vi "random_bit_sequence.vi"(11 "Length":i32) -> (3 "Bit Sequence":i8[](array[numeric]))   [LabVIEW 2012]
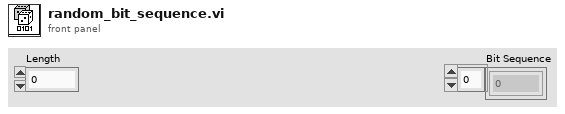
[diagram p1: front panel]
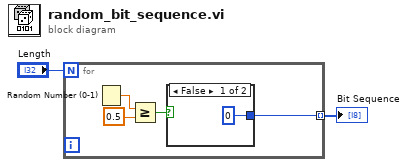
[diagram p0: block diagram]
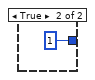
[diagram p2: hidden frame]
diagram:
  n1 = for {
    N: "Length" -> [_]
    tunnel: [w3] -> w1 mode=indexing
    n2 = Random Number (0-1)() -> (number: 0 to 1=w5:dbl)
    n3 = Greater Or Equal?(x=w5, y=0.5) -> (x >= y?=w4:bool)
    n4 = case shown="False" w4 {
      tunnel: [i8 0 i8 1] -> w3
      frame False {
      }
      frame True {
      }
    }
  }
  "Bit Sequence" <- w1
